vi "PYTHON VI Tree.vi"() -> ()   [LabVIEW 2009]
uses:
  PYTHON Session Refnum.ctl
panel:
  out "Python Session":T1
  # "PYTHON VI Tree.vi\n\nAn overview of all user functions from the Python VI Library\n\nCopyright (C) 2002 Rolf Kalbermatter rolf.kalbermatter@citeng.com\nCopyright (C) 2002 James Kring jim@jimkring.com\n\nPlease visit http://www.OpenG.org to learn about the\nOpen Source LabVIEW software movement.\n\nThis library is free software; you can redistribute it and/or\nmodify it under the terms of the GNU Lesser General Public\nLicense as published by the Free Software Foundation; either\nversion 2.1 of the License, or (at your option) any later version.\nThis library is distributed in the hope that it will be useful,\nbut WITHOUT ANY WARRANTY; without even the implied warranty of\nMERCHANTABILITY or FITNESS FOR A PARTICULAR PURPOSE. See the GNU\nLesser General Public License for more details.\nYou should have received a copy of the GNU Lesser General Public\nLicense along with this library; if not, write to the Free Software\nFoundation, Inc., 59 Temple Place, Suite 330, Boston, MA 02111-1307 USA"
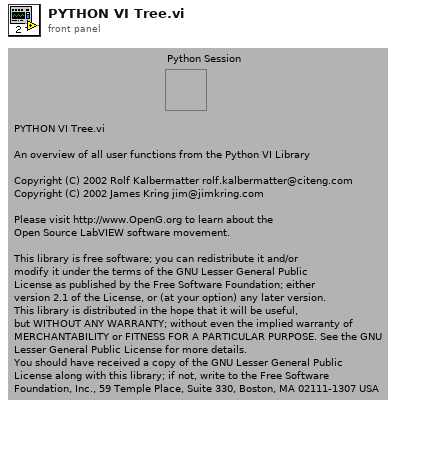
[diagram p1: front panel]
types:
  T1 = typedef "PYTHON Session Refnum.ctl" = refnum<k1>
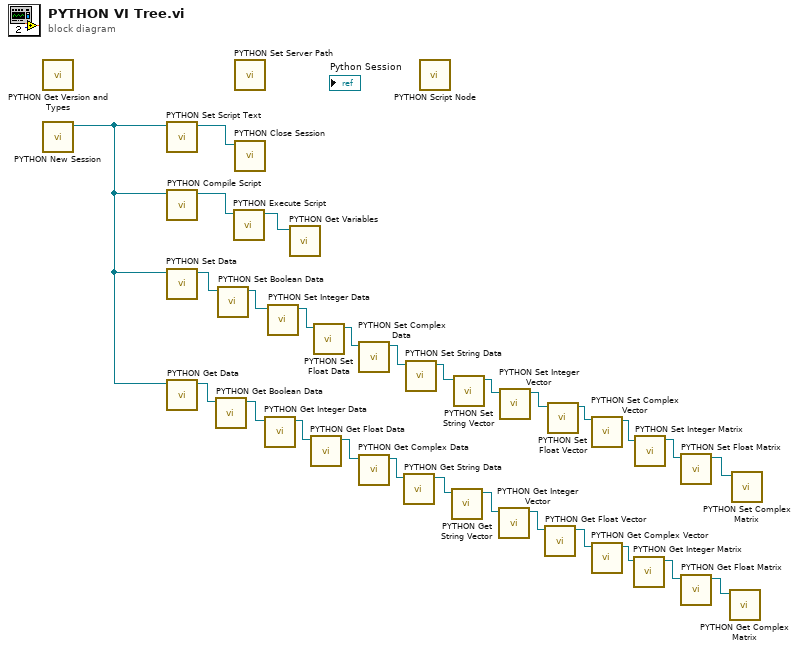
[diagram p0: block diagram]
diagram:
  n1 = call "PYTHON Get Version and Types.vi"() -> ()  [unwired: 5 in, 3 out]
  n2 = call "PYTHON New Session.vi"() -> ("Python Session"=w22:T1)  [unwired: 6 in, 1 out]
  n3 = call "PYTHON Set Script Text.vi"("Python Session in"=w22) -> ("Python Session out"=w28:T1)  [unwired: 5 in, 1 out]
  n4 = call "PYTHON Compile Script.vi"("Python Session in"=w22) -> ("Python Session out"=w23:T1)  [unwired: 5 in, 1 out]
  n5 = call-poly "PYTHON Set Data.vi"("Python Session in"=w22) -> ("Python Session out"=w27:T1)  [unwired: 5 in, 1 out]
  n6 = call-poly "PYTHON Get Data.vi"("Python Session in"=w22) -> ("Python Session out"=w17:T1)  [unwired: 4 in, 2 out]
  n7 = call "PYTHON Get Boolean Data.vi"("Python Session in"=w17) -> ("Python Session out"=w16:T1)  [unwired: 4 in, 2 out]
  n8 = call "PYTHON Set Boolean Data.vi"("Python Session in"=w27) -> ("Python Session out"=w15:T1)  [unwired: 5 in, 1 out]
  n9 = call "PYTHON Execute Script.vi"("Python Session in"=w23) -> ("Python Session out"=w18:T1)  [unwired: 5 in, 1 out]
  n10 = call "PYTHON Set Server Path.vi"() -> ()  [unwired: 7 in, 1 out]
  n11 = call "PYTHON Close Session.vi"("Python Session in"=w28) -> ()  [unwired: 6 in, 1 out]
  n12 = call "PYTHON Get Integer Data.vi"("Python Session in"=w16) -> ("Python Session out"=w21:T1)  [unwired: 4 in, 2 out]
  n13 = call "PYTHON Set Integer Data.vi"("Python Session in"=w15) -> ("Python Session out"=w26:T1)  [unwired: 5 in, 1 out]
  n14 = call "PYTHON Get Variables.vi"("Python Session in"=w18) -> ()  [unwired: 3 in, 4 out]
  n15 = call "PYTHON Get Float Data.vi"("Python Session in"=w21) -> ("Python Session out"=w20:T1)  [unwired: 4 in, 2 out]
  n16 = call "PYTHON Set Float Data.vi"("Python Session in"=w26) -> ("Python Session out"=w25:T1)  [unwired: 5 in, 1 out]
  n17 = call "PYTHON Set Complex Data.vi"("Python Session in"=w25) -> ("Python Session out"=w24:T1)  [unwired: 5 in, 1 out]
  n18 = call "PYTHON Get Complex Data.vi"("Python Session in"=w20) -> ("Python Session out"=w19:T1)  [unwired: 4 in, 2 out]
  n19 = call "PYTHON Get String Data.vi"("Python Session in"=w19) -> ("Python Session out"=w4:T1)  [unwired: 4 in, 2 out]
  n20 = call "PYTHON Set String Data.vi"("Python Session in"=w24) -> ("Python Session out"=w2:T1)  [unwired: 5 in, 1 out]
  n21 = call "PYTHON Script Node.vi"() -> ()  [unwired: 1 in]
  n22 = call "PYTHON Get String Vector.vi"("Python Session in"=w4) -> ("Python Session out"=w3:T1)  [unwired: 4 in, 2 out]
  n23 = call "PYTHON Set String Vector.vi"("Python Session in"=w2) -> ("Python Session out"=w1:T1)  [unwired: 5 in, 1 out]
  n24 = call "PYTHON Get Integer Vector.vi"("Python Session in"=w3) -> ("Python Session out"=w14:T1)  [unwired: 4 in, 2 out]
  n25 = call "PYTHON Set Integer Vector.vi"("Python Session in"=w1) -> ("Python Session out"=w9:T1)  [unwired: 5 in, 1 out]
  n26 = call "PYTHON Get Float Vector.vi"("Python Session in"=w14) -> ("Python Session out"=w13:T1)  [unwired: 4 in, 2 out]
  n27 = call "PYTHON Set Float Vector.vi"("Python Session in"=w9) -> ("Python Session out"=w8:T1)  [unwired: 5 in, 1 out]
  n28 = call "PYTHON Set Complex Vector.vi"("Python Session in"=w8) -> ("Python Session out"=w7:T1)  [unwired: 5 in, 1 out]
  n29 = call "PYTHON Get Complex Vector.vi"("Python Session in"=w13) -> ("Python Session out"=w12:T1)  [unwired: 4 in, 2 out]
  n30 = call "PYTHON Get Integer Matrix.vi"("Python Session in"=w12) -> ("Python Session out"=w11:T1)  [unwired: 4 in, 2 out]
  n31 = call "PYTHON Set Integer Matrix.vi"("Python Session in"=w7) -> ("Python Session out"=w6:T1)  [unwired: 5 in, 1 out]
  n32 = call "PYTHON Set Float Matrix.vi"("Python Session in"=w6) -> ("Python Session out"=w5:T1)  [unwired: 5 in, 1 out]
  n33 = call "PYTHON Get Float Matrix.vi"("Python Session in"=w11) -> ("Python Session out"=w10:T1)  [unwired: 4 in, 2 out]
  n34 = call "PYTHON Get Complex Matrix.vi"("Python Session in"=w10) -> ()  [unwired: 4 in, 3 out]
  n35 = call "PYTHON Set Complex Matrix.vi"("Python Session in"=w5) -> ()  [unwired: 5 in, 2 out]
